vi "ALinFramwork Controls.vi"() -> ()   [LabVIEW 2020]
panel:
  in  "Close":bool
  in  "图片下拉列表":u16(ring)
  in  "Launch":bool
  in  "Graph 2":bool
  in  "Graph":bool
  in  "Show 2":bool
  in  "Monitor":bool
  in  "UD":bool
  in  "LR":bool
  in  "Log":bool
  out "Help2":bool
  in  "Help":bool
  in  "Set":bool
  in  "Mode":bool
  in  "Set":bool
  in  "Copy":bool
  in  "C1":bool
  in  "Send":bool
  in  "Max":bool
  in  "LV":bool
  in  "SIE":bool
  in  "IMP":bool
  in  "Valve":bool
  in  "Manual":bool
  in  "Refresh":bool
  out "Warning":bool
  out "Reset":bool
  out "Connect":bool
  out "Start":bool
  out "LMG01":bool
  out "LMG01":bool
  out "Show":bool
  out "Valve":bool
  out "Pump":bool
  in  "Export":bool
  in  "Edit":bool
  in  "Release":bool
  in  "AF":bool
  in  "Search":bool
  in  "Import":bool
  in  "Delete":bool
  in  "Add":bool
  in  "C2":bool
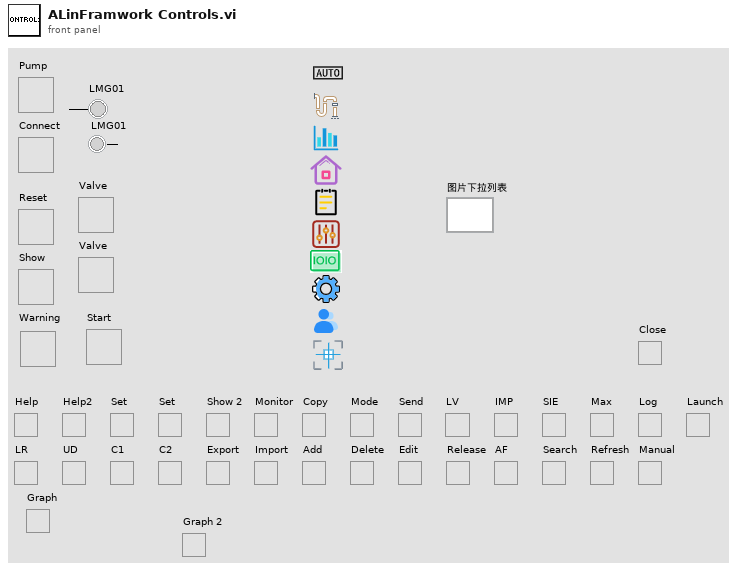
[diagram p1: front panel]
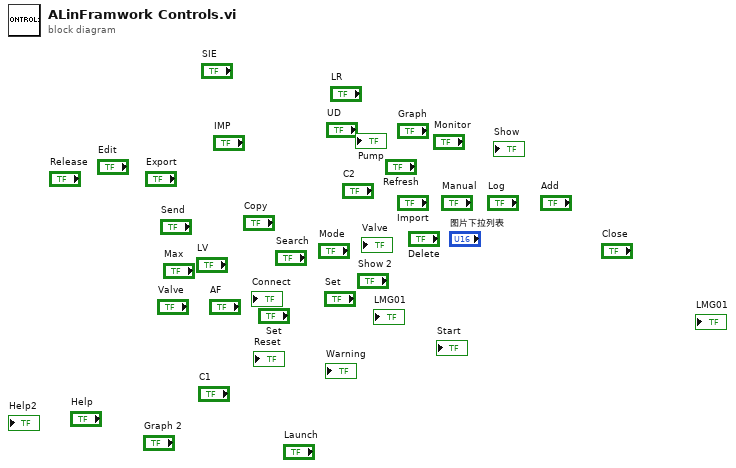
[diagram p0: block diagram]
diagram:
